vi "Write Base Path.vi"(8 "error in (no error)":errorcluster, 10 "HHP Path":path, 11 "CHM Generator in":refnum<class "CHM Generator.lvclass">) -> (0 "error out":errorcluster, 3 "CHM Generator out":refnum<class "CHM Generator.lvclass">)   [LabVIEW 2015]
uses:
  CHM Generator.lvclass
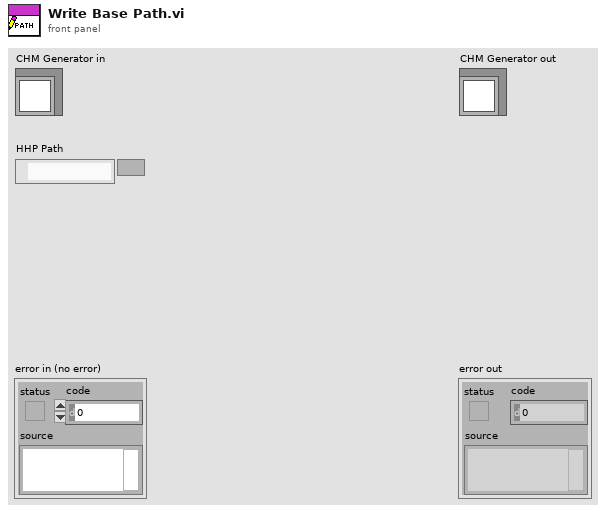
[diagram p1: front panel]
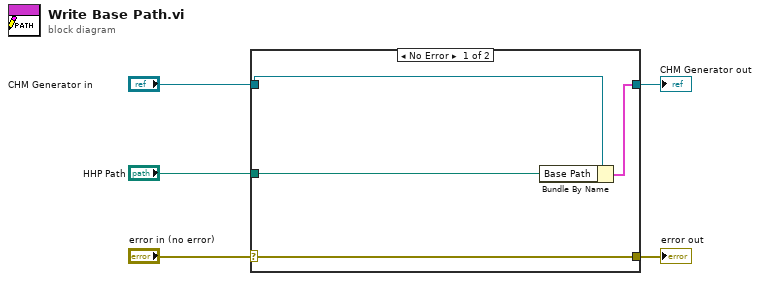
[diagram p0: block diagram]
diagram:
  n1 = case shown="No Error" "error in (no error)" {
    selector: "error in (no error)" -> [w9 w10]
    tunnel: [w9 w10] -> w4
    tunnel: [w7 w11] -> w2
    tunnel: "CHM Generator in" -> [w8 w11]
    tunnel: "HHP Path" -> [w6 _]
    frame No Error {
      n2 = Bundle By Name(cluster=w8, "Base Path"=w6) -> (w7:cluster{})
    }
    frame Error {
    }
  }
  "error out" <- w4
  "CHM Generator out" <- w2
